vi "Lab Panel V4.87.vi"() -> ()   [LabVIEW 2013] (continued)
                      tunnel: w2786 -> [_ w2799]
                      tunnel: w2785 -> [_ w2798]
                      tunnel: w2784 -> [_ w2797]
                      frame False {
                      }
                      frame True {
                        n1475 = stacked-sequence {
                          tunnel: w2804 -> [w2808 _ _]
                          tunnel: w2803 -> [_ w2810 _]
                          tunnel: w2802 -> [_ _ _]
                          tunnel: w2801 -> [_ _ w2816]
                          tunnel: w2800 -> [_ _ w2815]
                          tunnel: w2799 -> [_ _ w2814]
                          tunnel: w2798 -> [_ _ w2813]
                          tunnel: w2797 -> [_ _ w2812]
                          frame #0 {
                            w2805 = FALSE
                            n1476 = local write "mail control"("END") -> ()
                            n1477 = Bundle(cluster=w2808) -> (w2807:T4)  [unwired: 3 in]
                            n1478 = local write "DISP LAB01-1"(w2807) -> ()
                            n1479 = local write "O/I  LAB01-1"(w2805) -> ()
                            n1480 = local write "run lab01-1"(w2805) -> ()
                            n1481 = local write "RUN LAB01-1"(w2805) -> ()
                          }
                          frame #1 {
                            n1482 = TDMS Close(11:w2810) -> (0:w2809:errorcluster)  [unwired: 1 in, 1 out]
                            n1483 = local write "data file error"(w2809) -> ()
                          }
                          frame #2 {
                            n1484 = stacked-sequence {
                              tunnel: "LAB01-1" -> [w2818 w2820 _]
                              tunnel: w2816 -> [_ w2826 _]
                              tunnel: w2815 -> [_ w2825 _]
                              tunnel: w2814 -> [_ w2824 _]
                              tunnel: w2813 -> [_ w2823 _]
                              tunnel: w2812 -> [_ w2822 _]
                              frame #0 {
                                n1485 = call "sub vi - defrag tdms v1.vi"("panel id"=w2818) -> ("error out"=w2817:errorcluster)  [unwired: 10 in]
                                n1486 = local write "data file error"(w2817) -> ()
                              }
                              frame #1 {
                                n1487 = Bundle("STATUS"=w2826, "OUT SERVER ADDRESS"=w2825, "FROM ACCOUNT"=w2824, "Mail Test File To:"=w2823, "Mail Test Fail"=w2822) -> (w2819:T25)  [unwired: 1 in]
                                n1488 = call "Save data file to network drive v3.vi"("Input Cluster"=w2819, "panel id"=w2820) -> ("network file save error"=w2821:errorcluster)  [unwired: 8 in, 1 out]
                                n1489 = local write "data file error"(w2821) -> ()
                              }
                              frame #2 {
                              }
                            }
                          }
                        }
                      }
                    }
                  }
                }
              }
              frame #1 {
                # "LAB01-2"
                n1490 = local read "run lab01-2"() -> (w2831:bool)
                n1491 = case shown="True" w2831 {
                  tunnel: w2830 -> [_ w2835]
                  tunnel: w2829 -> [_ w2834]
                  tunnel: w2828 -> [_ w2833]
                  tunnel: w2827 -> [_ w2832]
                  frame False {
                  }
                  frame True {
                    n1492 = local read "DISP LAB01-2"() -> (w2843:T4)
                    n1493 = local read "TDMS LAB01-2"() -> (w2842:refnum<k34>)
                    n1494 = Unbundle(w2843) -> ("CYCLE"=w2837:dbl, "STATUS"=w2836:string)  [unwired: 1 out]
                    n1495 = Not Equal?(x=w2836, y="RUN") -> (x != y?=w2839:bool)
                    n1496 = Greater?(x=w2837, y=2.0) -> (0:w2840:bool)
                    n1497 = And(x=w2840, y=w2839) -> (x .and. y?=w2838:bool)
                    n1498 = case shown="True" w2838 {
                      tunnel: w2843 -> [_ w2852]
                      tunnel: w2842 -> [_ w2851]
                      tunnel: w2837 -> [_ w2850]
                      tunnel: w2836 -> [_ w2849]
                      tunnel: w2835 -> [_ w2848]
                      tunnel: w2834 -> [_ w2847]
                      tunnel: w2833 -> [_ w2846]
                      tunnel: w2832 -> [_ w2845]
                      frame False {
                      }
                      frame True {
                        n1499 = stacked-sequence {
                          tunnel: w2852 -> [w2855 _ _]
                          tunnel: w2851 -> [_ w2857 _]
                          tunnel: w2850 -> [_ _ _]
                          tunnel: w2849 -> [_ _ w2863]
                          tunnel: w2848 -> [_ _ w2862]
                          tunnel: w2847 -> [_ _ w2861]
                          tunnel: w2846 -> [_ _ w2860]
                          tunnel: w2845 -> [_ _ w2859]
                          frame #0 {
                            w2853 = FALSE
                            n1500 = local write "mail control"("END") -> ()
                            n1501 = Bundle(cluster=w2855) -> (w2856:T4)  [unwired: 3 in]
                            n1502 = local write "RUN LAB01-2"(w2853) -> ()
                            n1503 = local write "run lab01-2"(w2853) -> ()
                            n1504 = local write "O/I  LAB01-2"(w2853) -> ()
                            n1505 = local write "DISP LAB01-2"(w2856) -> ()
                          }
                          frame #1 {
                            n1506 = TDMS Close(11:w2857) -> (0:w2858:errorcluster)  [unwired: 1 in, 1 out]
                            n1507 = local write "data file error"(w2858) -> ()
                          }
                          frame #2 {
                            n1508 = stacked-sequence {
                              tunnel: "LAB01-2" -> [w2866 w2867]
                              tunnel: w2863 -> [_ w2872]
                              tunnel: w2862 -> [_ w2871]
                              tunnel: w2861 -> [_ w2870]
                              tunnel: w2860 -> [_ w2869]
                              tunnel: w2859 -> [_ w2868]
                              frame #0 {
                                n1509 = call "sub vi - defrag tdms v1.vi"("panel id"=w2866) -> ("error out"=w2865:errorcluster)  [unwired: 10 in]
                                n1510 = local write "data file error"(w2865) -> ()
                              }
                              frame #1 {
                                n1511 = Bundle("STATUS"=w2872, "OUT SERVER ADDRESS"=w2871, "FROM ACCOUNT"=w2870, "Mail Test File To:"=w2869, "Mail Test Fail"=w2868) -> (w2874:T25)  [unwired: 1 in]
                                n1512 = call "Save data file to network drive v3.vi"("Input Cluster"=w2874, "panel id"=w2867) -> ("network file save error"=w2873:errorcluster)  [unwired: 8 in, 1 out]
                                n1513 = local write "data file error"(w2873) -> ()
                              }
                            }
                          }
                        }
                      }
                    }
                  }
                }
              }
              frame #2 {
                # "LAB02-1"
                n1514 = local read "run lab02-1"() -> (w2879:bool)
                n1515 = case shown="True" w2879 {
                  tunnel: w2878 -> [_ w2883]
                  tunnel: w2877 -> [_ w2882]
                  tunnel: w2876 -> [_ w2881]
                  tunnel: w2875 -> [_ w2880]
                  frame False {
                  }
                  frame True {
                    n1516 = local read "DISP LAB02-1"() -> (w2891:T4)
                    n1517 = Unbundle(w2891) -> ("CYCLE"=w2887:dbl, "STATUS"=w2884:string)  [unwired: 1 out]
                    n1518 = local read "TDMS LAB02-1"() -> (w2890:refnum<k34>)
                    n1519 = Not Equal?(x=w2884, y="RUN") -> (x != y?=w2886:bool)
                    n1520 = Greater?(x=w2887, y=2.0) -> (0:w2888:bool)
                    n1521 = And(x=w2888, y=w2886) -> (x .and. y?=w2885:bool)
                    n1522 = case shown="True" w2885 {
                      tunnel: w2891 -> [_ w2899]
                      tunnel: w2890 -> [_ w2898]
                      tunnel: w2884 -> [_ w2897]
                      tunnel: w2883 -> [_ w2896]
                      tunnel: w2882 -> [_ w2895]
                      tunnel: w2881 -> [_ w2894]
                      tunnel: w2880 -> [_ w2893]
                      frame False {
                      }
                      frame True {
                        n1523 = stacked-sequence {
                          tunnel: w2899 -> [w2902 _ _]
                          tunnel: w2898 -> [_ w2904 _]
                          tunnel: w2897 -> [_ _ w2910]
                          tunnel: w2896 -> [_ _ w2909]
                          tunnel: w2895 -> [_ _ w2908]
                          tunnel: w2894 -> [_ _ w2907]
                          tunnel: w2893 -> [_ _ w2906]
                          frame #0 {
                            w2900 = FALSE
                            n1524 = local write "mail control"("END") -> ()
                            n1525 = Bundle(cluster=w2902) -> (w2903:T4)  [unwired: 3 in]
                            n1526 = local write "O/I  LAB02-1"(w2900) -> ()
                            n1527 = local write "RUN LAB02-1"(w2900) -> ()
                            n1528 = local write "run lab02-1"(w2900) -> ()
                            n1529 = local write "DISP LAB02-1"(w2903) -> ()
                          }
                          frame #1 {
                            n1530 = TDMS Close(11:w2904) -> (0:w2905:errorcluster)  [unwired: 1 in, 1 out]
                            n1531 = local write "data file error"(w2905) -> ()
                          }
                          frame #2 {
                            n1532 = stacked-sequence {
                              tunnel: "LAB02-1" -> [w2913 w2920]
                              tunnel: w2910 -> [_ w2918]
                              tunnel: w2909 -> [_ w2917]
                              tunnel: w2908 -> [_ w2916]
                              tunnel: w2907 -> [_ w2915]
                              tunnel: w2906 -> [_ w2914]
                              frame #0 {
                                n1533 = call "sub vi - defrag tdms v1.vi"("panel id"=w2913) -> ("error out"=w2912:errorcluster)  [unwired: 10 in]
                                n1534 = local write "data file error"(w2912) -> ()
                              }
                              frame #1 {
                                n1535 = Bundle("STATUS"=w2918, "OUT SERVER ADDRESS"=w2917, "FROM ACCOUNT"=w2916, "Mail Test File To:"=w2915, "Mail Test Fail"=w2914) -> (w2919:T25)  [unwired: 1 in]
                                n1536 = call "Save data file to network drive v3.vi"("Input Cluster"=w2919, "panel id"=w2920) -> ("network file save error"=w2921:errorcluster)  [unwired: 8 in, 1 out]
                                n1537 = local write "data file error"(w2921) -> ()
                              }
                            }
                          }
                        }
                      }
                    }
                  }
                }
              }
              frame #3 {
                # "LAB02-2"
                n1538 = local read "run lab02-2"() -> (w2926:bool)
                n1539 = case shown="True" w2926 {
                  tunnel: w2925 -> [_ w2930]
                  tunnel: w2924 -> [_ w2929]
                  tunnel: w2923 -> [_ w2928]
                  tunnel: w2922 -> [_ w2927]
                  frame False {
                  }
                  frame True {
                    n1540 = local read "DISP LAB02-2"() -> (w2938:T4)
                    n1541 = local read "TDMS LAB02-2"() -> (w2937:refnum<k34>)
                    n1542 = Unbundle(w2938) -> ("CYCLE"=w2934:dbl, "STATUS"=w2931:string)  [unwired: 1 out]
                    n1543 = Not Equal?(x=w2931, y="RUN") -> (x != y?=w2933:bool)
                    n1544 = Greater?(x=w2934, y=2.0) -> (0:w2935:bool)
                    n1545 = And(x=w2935, y=w2933) -> (x .and. y?=w2932:bool)
                    n1546 = case shown="True" w2932 {
                      tunnel: w2938 -> [_ w2946]
                      tunnel: w2937 -> [_ w2945]
                      tunnel: w2931 -> [_ w2944]
                      tunnel: w2930 -> [_ w2943]
                      tunnel: w2929 -> [_ w2942]
                      tunnel: w2928 -> [_ w2941]
                      tunnel: w2927 -> [_ w2940]
                      frame False {
                      }
                      frame True {
                        n1547 = stacked-sequence {
                          tunnel: w2946 -> [w2949 _ _]
                          tunnel: w2945 -> [_ w2951 _]
                          tunnel: w2944 -> [_ _ w2957]
                          tunnel: w2943 -> [_ _ w2956]
                          tunnel: w2942 -> [_ _ w2955]
                          tunnel: w2941 -> [_ _ w2954]
                          tunnel: w2940 -> [_ _ w2953]
                          frame #0 {
                            w2947 = FALSE
                            n1548 = local write "mail control"("END") -> ()
                            n1549 = Bundle(cluster=w2949) -> (w2950:T4)  [unwired: 3 in]
                            n1550 = local write "O/I  LAB02-2"(w2947) -> ()
                            n1551 = local write "run lab02-2"(w2947) -> ()
                            n1552 = local write "RUN LAB02-2"(w2947) -> ()
                            n1553 = local write "DISP LAB02-2"(w2950) -> ()
                          }
                          frame #1 {
                            n1554 = TDMS Close(11:w2951) -> (0:w2952:errorcluster)  [unwired: 1 in, 1 out]
                            n1555 = local write "data file error"(w2952) -> ()
                          }
                          frame #2 {
                            n1556 = stacked-sequence {
                              tunnel: "LAB02-2" -> [w2960 w2966]
                              tunnel: w2957 -> [_ w2965]
                              tunnel: w2956 -> [_ w2964]
                              tunnel: w2955 -> [_ w2963]
                              tunnel: w2954 -> [_ w2962]
                              tunnel: w2953 -> [_ w2961]
                              frame #0 {
                                n1557 = call "sub vi - defrag tdms v1.vi"("panel id"=w2960) -> ("error out"=w2959:errorcluster)  [unwired: 10 in]
                                n1558 = local write "data file error"(w2959) -> ()
                              }
                              frame #1 {
                                n1559 = Bundle("STATUS"=w2965, "OUT SERVER ADDRESS"=w2964, "FROM ACCOUNT"=w2963, "Mail Test File To:"=w2962, "Mail Test Fail"=w2961) -> (w2968:T25)  [unwired: 1 in]
                                n1560 = call "Save data file to network drive v3.vi"("Input Cluster"=w2968, "panel id"=w2966) -> ("network file save error"=w2967:errorcluster)  [unwired: 8 in, 1 out]
                                n1561 = local write "data file error"(w2967) -> ()
                              }
                            }
                          }
                        }
                      }
                    }
                  }
                }
              }
              frame #4 {
                # "LAB03-1"
                n1562 = local read "run lab03-1"() -> (w2973:bool)
                n1563 = case shown="True" w2973 {
                  tunnel: w2972 -> [_ w2977]
                  tunnel: w2971 -> [_ w2976]
                  tunnel: w2970 -> [_ w2975]
                  tunnel: w2969 -> [_ w2974]
                  frame False {
                  }
                  frame True {
                    n1564 = local read "DISP LAB03-1"() -> (w2985:T4)
                    n1565 = local read "TDMS LAB03-1"() -> (w2984:refnum<k34>)
                    n1566 = Unbundle(w2985) -> ("CYCLE"=w2981:dbl, "STATUS"=w2978:string)  [unwired: 1 out]
                    n1567 = Not Equal?(x=w2978, y="RUN") -> (x != y?=w2980:bool)
                    n1568 = Greater?(x=w2981, y=2.0) -> (0:w2982:bool)
                    n1569 = And(x=w2982, y=w2980) -> (x .and. y?=w2979:bool)
                    n1570 = case shown="True" w2979 {
                      tunnel: w2985 -> [_ w2993]
                      tunnel: w2984 -> [_ w2992]
                      tunnel: w2978 -> [_ w2991]
                      tunnel: w2977 -> [_ w2990]
                      tunnel: w2976 -> [_ w2989]
                      tunnel: w2975 -> [_ w2988]
                      tunnel: w2974 -> [_ w2987]
                      frame False {
                      }
                      frame True {
                        n1571 = stacked-sequence {
                          tunnel: w2993 -> [w2996 _ _]
                          tunnel: w2992 -> [_ w2998 _]
                          tunnel: w2991 -> [_ _ w3004]
                          tunnel: w2990 -> [_ _ w3003]
                          tunnel: w2989 -> [_ _ w3002]
                          tunnel: w2988 -> [_ _ w3001]
                          tunnel: w2987 -> [_ _ w3000]
                          frame #0 {
                            w2994 = FALSE
                            n1572 = local write "mail control"("END") -> ()
                            n1573 = Bundle(cluster=w2996) -> (w2997:T4)  [unwired: 3 in]
                            n1574 = local write "O/I  LAB03-1"(w2994) -> ()
                            n1575 = local write "run lab03-1"(w2994) -> ()
                            n1576 = local write "RUN LAB03-1"(w2994) -> ()
                            n1577 = local write "DISP LAB03-1"(w2997) -> ()
                          }
                          frame #1 {
                            n1578 = TDMS Close(11:w2998) -> (0:w2999:errorcluster)  [unwired: 1 in, 1 out]
                            n1579 = local write "data file error"(w2999) -> ()
                          }
                          frame #2 {
                            n1580 = stacked-sequence {
                              tunnel: "LAB03-1" -> [w3007 w3013]
                              tunnel: w3004 -> [_ w3012]
                              tunnel: w3003 -> [_ w3011]
                              tunnel: w3002 -> [_ w3010]
                              tunnel: w3001 -> [_ w3009]
                              tunnel: w3000 -> [_ w3008]
                              frame #0 {
                                n1581 = call "sub vi - defrag tdms v1.vi"("panel id"=w3007) -> ("error out"=w3006:errorcluster)  [unwired: 10 in]
                                n1582 = local write "data file error"(w3006) -> ()
                              }
                              frame #1 {
                                n1583 = Bundle("STATUS"=w3012, "OUT SERVER ADDRESS"=w3011, "FROM ACCOUNT"=w3010, "Mail Test File To:"=w3009, "Mail Test Fail"=w3008) -> (w3015:T25)  [unwired: 1 in]
                                n1584 = call "Save data file to network drive v3.vi"("Input Cluster"=w3015, "panel id"=w3013) -> ("network file save error"=w3014:errorcluster)  [unwired: 8 in, 1 out]
                                n1585 = local write "data file error"(w3014) -> ()
                              }
                            }
                          }
                        }
                      }
                    }
                  }
                }
              }
              frame #5 {
                # "LAB03-2"
                n1586 = local read "run lab03-2"() -> (w3020:bool)
                n1587 = case shown="True" w3020 {
                  tunnel: w3019 -> [_ w3024]
                  tunnel: w3018 -> [_ w3023]
                  tunnel: w3017 -> [_ w3022]
                  tunnel: w3016 -> [_ w3021]
                  frame False {
                  }
                  frame True {
                    n1588 = local read "DISP LAB03-2"() -> (w3032:T4)
                    n1589 = Unbundle(w3032) -> ("CYCLE"=w3028:dbl, "STATUS"=w3025:string)  [unwired: 1 out]
                    n1590 = local read "TDMS LAB03-2"() -> (w3031:refnum<k34>)
                    n1591 = Not Equal?(x=w3025, y="RUN") -> (x != y?=w3027:bool)
                    n1592 = Greater?(x=w3028, y=2.0) -> (0:w3029:bool)
                    n1593 = And(x=w3029, y=w3027) -> (x .and. y?=w3026:bool)
                    n1594 = case shown="True" w3026 {
                      tunnel: w3032 -> [_ w3040]
                      tunnel: w3031 -> [_ w3039]
                      tunnel: w3025 -> [_ w3038]
                      tunnel: w3024 -> [_ w3037]
                      tunnel: w3023 -> [_ w3036]
                      tunnel: w3022 -> [_ w3035]
                      tunnel: w3021 -> [_ w3034]
                      frame False {
                      }
                      frame True {
                        n1595 = stacked-sequence {
                          tunnel: w3040 -> [w3043 _ _]
                          tunnel: w3039 -> [_ w3045 _]
                          tunnel: w3038 -> [_ _ w3051]
                          tunnel: w3037 -> [_ _ w3050]
                          tunnel: w3036 -> [_ _ w3049]
                          tunnel: w3035 -> [_ _ w3048]
                          tunnel: w3034 -> [_ _ w3047]
                          frame #0 {
                            w3041 = FALSE
                            n1596 = local write "mail control"("END") -> ()
                            n1597 = Bundle(cluster=w3043) -> (w3044:T4)  [unwired: 3 in]
                            n1598 = local write "RUN LAB03-2"(w3041) -> ()
                            n1599 = local write "O/I  LAB03-2"(w3041) -> ()
                            n1600 = local write "DISP LAB03-2"(w3044) -> ()
                            n1601 = local write "run lab03-2"(w3041) -> ()
                          }
                          frame #1 {
                            n1602 = TDMS Close(11:w3045) -> (0:w3046:errorcluster)  [unwired: 1 in, 1 out]
                            n1603 = local write "data file error"(w3046) -> ()
                          }
                          frame #2 {
                            n1604 = stacked-sequence {
                              tunnel: "LAB03-2" -> [w3054 w3055]
                              tunnel: w3051 -> [_ w3060]
                              tunnel: w3050 -> [_ w3059]
                              tunnel: w3049 -> [_ w3058]
                              tunnel: w3048 -> [_ w3057]
                              tunnel: w3047 -> [_ w3056]
                              frame #0 {
                                n1605 = call "sub vi - defrag tdms v1.vi"("panel id"=w3054) -> ("error out"=w3053:errorcluster)  [unwired: 10 in]
                                n1606 = local write "data file error"(w3053) -> ()
                              }
                              frame #1 {
                                n1607 = Bundle("STATUS"=w3060, "OUT SERVER ADDRESS"=w3059, "FROM ACCOUNT"=w3058, "Mail Test File To:"=w3057, "Mail Test Fail"=w3056) -> (w3062:T25)  [unwired: 1 in]
                                n1608 = call "Save data file to network drive v3.vi"("Input Cluster"=w3062, "panel id"=w3055) -> ("network file save error"=w3061:errorcluster)  [unwired: 8 in, 1 out]
                                n1609 = local write "data file error"(w3061) -> ()
                              }
                            }
                          }
                        }
                      }
                    }
                  }
                }
              }
              frame #6 {
                # "LAB04-1"
                n1610 = local read "run lab04-1"() -> (w3067:bool)
                n1611 = case shown="True" w3067 {
                  tunnel: w3066 -> [_ w3071]
                  tunnel: w3065 -> [_ w3070]
                  tunnel: w3064 -> [_ w3069]
                  tunnel: w3063 -> [_ w3068]
                  frame False {
                  }
                  frame True {
                    n1612 = local read "DISP LAB04-1"() -> (w3079:T4)
                    n1613 = Unbundle(w3079) -> ("CYCLE"=w3075:dbl, "STATUS"=w3072:string)  [unwired: 1 out]
                    n1614 = local read "TDMS LAB04-1"() -> (w3078:refnum<k34>)
                    n1615 = Not Equal?(x=w3072, y="RUN") -> (x != y?=w3074:bool)
                    n1616 = Greater?(x=w3075, y=2.0) -> (0:w3076:bool)
                    n1617 = And(x=w3076, y=w3074) -> (x .and. y?=w3073:bool)
                    n1618 = case shown="True" w3073 {
                      tunnel: w3079 -> [_ w3087]
                      tunnel: w3078 -> [_ w3086]
                      tunnel: w3072 -> [_ w3085]
                      tunnel: w3071 -> [_ w3084]
                      tunnel: w3070 -> [_ w3083]
                      tunnel: w3069 -> [_ w3082]
                      tunnel: w3068 -> [_ w3081]
                      frame False {
                      }
                      frame True {
                        n1619 = stacked-sequence {
                          tunnel: w3087 -> [w3090 _ _]
                          tunnel: w3086 -> [_ w3092 _]
                          tunnel: w3085 -> [_ _ w3098]
                          tunnel: w3084 -> [_ _ w3097]
                          tunnel: w3083 -> [_ _ w3096]
                          tunnel: w3082 -> [_ _ w3095]
                          tunnel: w3081 -> [_ _ w3094]
                          frame #0 {
                            w3088 = FALSE
                            n1620 = local write "mail control"("END") -> ()
                            n1621 = Bundle(cluster=w3090) -> (w3091:T4)  [unwired: 3 in]
                            n1622 = local write "RUN LAB04-1"(w3088) -> ()
                            n1623 = local write "O/I  LAB04-1"(w3088) -> ()
                            n1624 = local write "run lab04-1"(w3088) -> ()
                            n1625 = local write "DISP LAB04-1"(w3091) -> ()
                          }
                          frame #1 {
                            n1626 = TDMS Close(11:w3092) -> (0:w3093:errorcluster)  [unwired: 1 in, 1 out]
                            n1627 = local write "data file error"(w3093) -> ()
                          }
                          frame #2 {
                            n1628 = stacked-sequence {
                              tunnel: "LAB04-1" -> [w3101 w3102]
                              tunnel: w3098 -> [_ w3107]
                              tunnel: w3097 -> [_ w3106]
                              tunnel: w3096 -> [_ w3105]
                              tunnel: w3095 -> [_ w3104]
                              tunnel: w3094 -> [_ w3103]
                              frame #0 {
                                n1629 = call "sub vi - defrag tdms v1.vi"("panel id"=w3101) -> ("error out"=w3100:errorcluster)  [unwired: 10 in]
                                n1630 = local write "data file error"(w3100) -> ()
                              }
                              frame #1 {
                                n1631 = Bundle("STATUS"=w3107, "OUT SERVER ADDRESS"=w3106, "FROM ACCOUNT"=w3105, "Mail Test File To:"=w3104, "Mail Test Fail"=w3103) -> (w3109:T25)  [unwired: 1 in]
                                n1632 = call "Save data file to network drive v3.vi"("Input Cluster"=w3109, "panel id"=w3102) -> ("network file save error"=w3108:errorcluster)  [unwired: 8 in, 1 out]
                                n1633 = local write "data file error"(w3108) -> ()
                              }
                            }
                          }
                        }
                      }
                    }
                  }
                }
              }
              frame #7 {
                # "LAB04-2"
                n1634 = local read "run lab04-2"() -> (w3114:bool)
                n1635 = case shown="True" w3114 {
                  tunnel: w3113 -> [_ w3118]
                  tunnel: w3112 -> [_ w3117]
                  tunnel: w3111 -> [_ w3116]
                  tunnel: w3110 -> [_ w3115]
                  frame False {
                  }
                  frame True {
                    n1636 = local read "DISP LAB04-2"() -> (w3126:T4)
                    n1637 = Unbundle(w3126) -> ("CYCLE"=w3122:dbl, "STATUS"=w3119:string)  [unwired: 1 out]
                    n1638 = Not Equal?(x=w3119, y="RUN") -> (x != y?=w3121:bool)
                    n1639 = local read "TDMS LAB04-2"() -> (w3125:refnum<k34>)
                    n1640 = Greater?(x=w3122, y=2.0) -> (0:w3123:bool)
                    n1641 = And(x=w3123, y=w3121) -> (x .and. y?=w3120:bool)
                    n1642 = case shown="True" w3120 {
                      tunnel: w3126 -> [_ w3134]
                      tunnel: w3125 -> [_ w3133]
                      tunnel: w3119 -> [_ w3132]
                      tunnel: w3118 -> [_ w3131]
                      tunnel: w3117 -> [_ w3130]
                      tunnel: w3116 -> [_ w3129]
                      tunnel: w3115 -> [_ w3128]
                      frame False {
                      }
                      frame True {
                        n1643 = stacked-sequence {
                          tunnel: w3134 -> [w3137 _ _]
                          tunnel: w3133 -> [_ w3139 _]
                          tunnel: w3132 -> [_ _ w3145]
                          tunnel: w3131 -> [_ _ w3144]
                          tunnel: w3130 -> [_ _ w3143]
                          tunnel: w3129 -> [_ _ w3142]
                          tunnel: w3128 -> [_ _ w3141]
                          frame #0 {
                            w3135 = FALSE
                            n1644 = local write "mail control"("END") -> ()
                            n1645 = Bundle(cluster=w3137) -> (w3138:T4)  [unwired: 3 in]
                            n1646 = local write "O/I  LAB04-2"(w3135) -> ()
                            n1647 = local write "RUN LAB04-2"(w3135) -> ()
                            n1648 = local write "run lab04-2"(w3135) -> ()
                            n1649 = local write "DISP LAB04-2"(w3138) -> ()
                          }
                          frame #1 {
                            n1650 = TDMS Close(11:w3139) -> (0:w3140:errorcluster)  [unwired: 1 in, 1 out]
                            n1651 = local write "data file error"(w3140) -> ()
                          }
                          frame #2 {
                            n1652 = stacked-sequence {
                              tunnel: "LAB04-2" -> [w3148 w3149]
                              tunnel: w3145 -> [_ w3154]
                              tunnel: w3144 -> [_ w3153]
                              tunnel: w3143 -> [_ w3152]
                              tunnel: w3142 -> [_ w3151]
                              tunnel: w3141 -> [_ w3150]
                              frame #0 {
                                n1653 = call "sub vi - defrag tdms v1.vi"("panel id"=w3148) -> ("error out"=w3147:errorcluster)  [unwired: 10 in]
                                n1654 = local write "data file error"(w3147) -> ()
                              }
                              frame #1 {
                                n1655 = Bundle("STATUS"=w3154, "OUT SERVER ADDRESS"=w3153, "FROM ACCOUNT"=w3152, "Mail Test File To:"=w3151, "Mail Test Fail"=w3150) -> (w3156:T25)  [unwired: 1 in]
                                n1656 = call "Save data file to network drive v3.vi"("Input Cluster"=w3156, "panel id"=w3149) -> ("network file save error"=w3155:errorcluster)  [unwired: 8 in, 1 out]
                                n1657 = local write "data file error"(w3155) -> ()
                              }
                            }
                          }
                        }
                      }
                    }
                  }
                }
              }
              frame #8 {
                # "LAB05-1"
                n1658 = local read "run lab05-1"() -> (w3161:bool)
                n1659 = case shown="True" w3161 {
                  tunnel: w3160 -> [_ w3165]
                  tunnel: w3159 -> [_ w3164]
                  tunnel: w3158 -> [_ w3163]
                  tunnel: w3157 -> [_ w3162]
                  frame False {
                  }
                  frame True {
                    n1660 = local read "DISP LAB05-1"() -> (w3173:T4)
                    n1661 = Unbundle(w3173) -> ("CYCLE"=w3169:dbl, "STATUS"=w3166:string)  [unwired: 1 out]
                    n1662 = Not Equal?(x=w3166, y="RUN") -> (x != y?=w3168:bool)
                    n1663 = local read "TDMS LAB05-1"() -> (w3172:refnum<k34>)
                    n1664 = Greater?(x=w3169, y=2.0) -> (0:w3170:bool)
                    n1665 = And(x=w3170, y=w3168) -> (x .and. y?=w3167:bool)
                    n1666 = case shown="True" w3167 {
                      tunnel: w3173 -> [_ w3181]
                      tunnel: w3172 -> [_ w3180]
                      tunnel: w3166 -> [_ w3179]
                      tunnel: w3165 -> [_ w3178]
                      tunnel: w3164 -> [_ w3177]
                      tunnel: w3163 -> [_ w3176]
                      tunnel: w3162 -> [_ w3175]
                      frame False {
                      }
                      frame True {
                        n1667 = stacked-sequence {
                          tunnel: w3181 -> [w3184 _ _]
                          tunnel: w3180 -> [_ w3186 _]
                          tunnel: w3179 -> [_ _ w3192]
                          tunnel: w3178 -> [_ _ w3191]
                          tunnel: w3177 -> [_ _ w3190]
                          tunnel: w3176 -> [_ _ w3189]
                          tunnel: w3175 -> [_ _ w3188]
                          frame #0 {
                            w3182 = FALSE
                            n1668 = local write "mail control"("END") -> ()
                            n1669 = Bundle(cluster=w3184) -> (w3185:T4)  [unwired: 3 in]
                            n1670 = local write "O/I  LAB05-1"(w3182) -> ()
                            n1671 = local write "RUN LAB05-1"(w3182) -> ()
                            n1672 = local write "run lab05-1"(w3182) -> ()
                            n1673 = local write "DISP LAB05-1"(w3185) -> ()
                          }
                          frame #1 {
                            n1674 = TDMS Close(11:w3186) -> (0:w3187:errorcluster)  [unwired: 1 in, 1 out]
                            n1675 = local write "data file error"(w3187) -> ()
                          }
                          frame #2 {
                            n1676 = stacked-sequence {
                              tunnel: "LAB05-1" -> [w3195 w3201]
                              tunnel: w3192 -> [_ w3200]
                              tunnel: w3191 -> [_ w3199]
                              tunnel: w3190 -> [_ w3198]
                              tunnel: w3189 -> [_ w3197]
                              tunnel: w3188 -> [_ w3196]
                              frame #0 {
                                n1677 = call "sub vi - defrag tdms v1.vi"("panel id"=w3195) -> ("error out"=w3194:errorcluster)  [unwired: 10 in]
                                n1678 = local write "data file error"(w3194) -> ()
                              }
                              frame #1 {
                                n1679 = Bundle("STATUS"=w3200, "OUT SERVER ADDRESS"=w3199, "FROM ACCOUNT"=w3198, "Mail Test File To:"=w3197, "Mail Test Fail"=w3196) -> (w3203:T25)  [unwired: 1 in]
                                n1680 = call "Save data file to network drive v3.vi"("Input Cluster"=w3203, "panel id"=w3201) -> ("network file save error"=w3202:errorcluster)  [unwired: 8 in, 1 out]
                                n1681 = local write "data file error"(w3202) -> ()
                              }
                            }
                          }
                        }
                      }
                    }
                  }
                }
              }
              frame #9 {
                # "LAB05-2"
                n1682 = local read "run lab05-2"() -> (w3208:bool)
                n1683 = case shown="True" w3208 {
                  tunnel: w3207 -> [_ w3212]
                  tunnel: w3206 -> [_ w3211]
                  tunnel: w3205 -> [_ w3210]
                  tunnel: w3204 -> [_ w3209]
                  frame False {
                  }
                  frame True {
                    n1684 = local read "DISP LAB05-2"() -> (w3220:T4)
                    n1685 = Unbundle(w3220) -> ("CYCLE"=w3216:dbl, "STATUS"=w3213:string)  [unwired: 1 out]
                    n1686 = Not Equal?(x=w3213, y="RUN") -> (x != y?=w3215:bool)
                    n1687 = local read "TDMS LAB05-2"() -> (w3219:refnum<k34>)
                    n1688 = Greater?(x=w3216, y=2.0) -> (0:w3217:bool)
                    n1689 = And(x=w3217, y=w3215) -> (x .and. y?=w3214:bool)
                    n1690 = case shown="True" w3214 {
                      tunnel: w3220 -> [_ w3228]
                      tunnel: w3219 -> [_ w3227]
                      tunnel: w3213 -> [_ w3226]
                      tunnel: w3212 -> [_ w3225]
                      tunnel: w3211 -> [_ w3224]
                      tunnel: w3210 -> [_ w3223]
                      tunnel: w3209 -> [_ w3222]
                      frame False {
                      }
                      frame True {
                        n1691 = stacked-sequence {
                          tunnel: w3228 -> [w3231 _ _]
                          tunnel: w3227 -> [_ w3233 _]
                          tunnel: w3226 -> [_ _ w3239]
                          tunnel: w3225 -> [_ _ w3238]
                          tunnel: w3224 -> [_ _ w3237]
                          tunnel: w3223 -> [_ _ w3236]
                          tunnel: w3222 -> [_ _ w3235]
                          frame #0 {
                            w3229 = FALSE
                            n1692 = local write "mail control"("END") -> ()
                            n1693 = Bundle(cluster=w3231) -> (w3232:T4)  [unwired: 3 in]
                            n1694 = local write "RUN LAB05-2"(w3229) -> ()
                            n1695 = local write "O/I  LAB05-2"(w3229) -> ()
                            n1696 = local write "run lab05-2"(w3229) -> ()
                            n1697 = local write "DISP LAB05-2"(w3232) -> ()
                          }
                          frame #1 {
                            n1698 = TDMS Close(11:w3233) -> (0:w3234:errorcluster)  [unwired: 1 in, 1 out]
                            n1699 = local write "data file error"(w3234) -> ()
                          }
                          frame #2 {
                            n1700 = stacked-sequence {
                              tunnel: "LAB05-2" -> [w3242 w3248]
                              tunnel: w3239 -> [_ w3247]
                              tunnel: w3238 -> [_ w3246]
                              tunnel: w3237 -> [_ w3245]
                              tunnel: w3236 -> [_ w3244]
                              tunnel: w3235 -> [_ w3243]
                              frame #0 {
                                n1701 = call "sub vi - defrag tdms v1.vi"("panel id"=w3242) -> ("error out"=w3241:errorcluster)  [unwired: 10 in]
                                n1702 = local write "data file error"(w3241) -> ()
                              }
                              frame #1 {
                                n1703 = Bundle("STATUS"=w3247, "OUT SERVER ADDRESS"=w3246, "FROM ACCOUNT"=w3245, "Mail Test File To:"=w3244, "Mail Test Fail"=w3243) -> (w3250:T25)  [unwired: 1 in]
                                n1704 = call "Save data file to network drive v3.vi"("Input Cluster"=w3250, "panel id"=w3248) -> ("network file save error"=w3249:errorcluster)  [unwired: 8 in, 1 out]
                                n1705 = local write "data file error"(w3249) -> ()
                              }
                            }
                          }
                        }
                      }
                    }
                  }
                }
              }
            }
            n1706 = local read "Network Directory"() -> (w2764:path)
            n1707 = global write "Global 1.vi" "Network Drive"(w2764) -> ()
          }
          frame #7 {
            # "disable functions"
            n1708 = stacked-sequence {
              tunnel: w3260 -> [w3274 _ w3331]
              tunnel: w3259 -> [w3269 _ w3330]
              tunnel: w3258 -> [w3268 _ w3329]
              tunnel: w3257 -> [w3266 _ w3328]
              tunnel: w3256 -> [w3267 _ w3327]
              tunnel: w3255 -> [_ w3291 w3326]
              tunnel: w3254 -> [_ w3292 w3325]
              tunnel: w3253 -> [_ w3293 w3324]
              tunnel: w3252 -> [_ w3294 w3323]
              tunnel: w3251 -> [_ w3295 w3322]
              frame #0 {
                n1709 = Select(t=2, s=w3266, f=0) -> (s? t:f=w3262:i32)
                n1710 = Select(t=2, s=w3268, f=0) -> (s? t:f=w3263:i32)
                n1711 = Select(t=2, s=w3267, f=0) -> (s? t:f=w3261:i32)
                n1712 = Select(t=2, s=w3274, f=0) -> (s? t:f=w3265:i32)
                n1713 = Select(t=2, s=w3269, f=0) -> (s? t:f=w3264:i32)
                n1714 = property on="SELECT LAB02-2" class="RadioBtnsControl (strict)"("DisabledEnum"=w3262) -> ()  [unwired: 2 in, 2 out]
                n1715 = property on="SELECT LAB02-1" class="RadioBtnsControl (strict)"("DisabledEnum"=w3263) -> ()  [unwired: 2 in, 2 out]
                n1716 = property on="SELECT LAB03-1" class="RadioBtnsControl (strict)"("DisabledEnum"=w3261) -> ()  [unwired: 2 in, 2 out]
                n1717 = property on="SELECT LAB01-1" class="RadioBtnsControl (strict)"("DisabledEnum"=w3265) -> ()  [unwired: 2 in, 2 out]
                n1718 = property on="SELECT LAB01-2" class="RadioBtnsControl (strict)"("DisabledEnum"=w3264) -> ()  [unwired: 2 in, 2 out]
                n1719 = Not(x=w3274) -> (.not. x?=w3275:bool)
                n1720 = property on="RESULT LAB01-1" class="Bool (strict)"("Visible"=w3275) -> ()  [unwired: 2 in, 2 out]
                n1721 = Not(x=w3269) -> (.not. x?=w3273:bool)
                n1722 = Not(x=w3268) -> (.not. x?=w3272:bool)
                n1723 = Not(x=w3266) -> (.not. x?=w3271:bool)
                n1724 = property on="RESULT LAB01-2" class="Bool (strict)"("Visible"=w3273) -> ()  [unwired: 2 in, 2 out]
                n1725 = Not(x=w3267) -> (.not. x?=w3270:bool)
                n1726 = property on="RESULT LAB02-1" class="Bool (strict)"("Visible"=w3272) -> ()  [unwired: 2 in, 2 out]
                n1727 = property on="RESULT LAB02-2" class="Bool (strict)"("Visible"=w3271) -> ()  [unwired: 2 in, 2 out]
                n1728 = property on="RESULT LAB03-1" class="Bool (strict)"("Visible"=w3270) -> ()  [unwired: 2 in, 2 out]
                n1729 = property on="SET LAB01-1" class="Clust (strict)"("DisabledEnum"=w3265) -> ()  [unwired: 2 in, 2 out]
                n1730 = property on="SET LAB01-2" class="Clust (strict)"("DisabledEnum"=w3264) -> ()  [unwired: 2 in, 2 out]
                n1731 = property on="SET LAB02-1" class="Clust (strict)"("DisabledEnum"=w3263) -> ()  [unwired: 2 in, 2 out]
                n1732 = property on="SET LAB02-2" class="Clust (strict)"("DisabledEnum"=w3262) -> ()  [unwired: 2 in, 2 out]
                n1733 = property on="SET LAB03-1" class="Clust (strict)"("DisabledEnum"=w3261) -> ()  [unwired: 2 in, 2 out]
                n1734 = property on="O/I  LAB01-1" class="Bool (strict)"("DisabledEnum"=w3265) -> ()  [unwired: 2 in, 2 out]
                n1735 = property on="O/I  LAB01-2" class="Bool (strict)"("DisabledEnum"=w3264) -> ()  [unwired: 2 in, 2 out]
                n1736 = property on="O/I  LAB02-1" class="Bool (strict)"("DisabledEnum"=w3263) -> ()  [unwired: 2 in, 2 out]
                n1737 = property on="O/I  LAB02-2" class="Bool (strict)"("DisabledEnum"=w3262) -> ()  [unwired: 2 in, 2 out]
                n1738 = property on="O/I  LAB03-1" class="Bool (strict)"("DisabledEnum"=w3261) -> ()  [unwired: 2 in, 2 out]
              }
              frame #1 {
                n1739 = Select(t=2, s=w3295, f=0) -> (s? t:f=w3286:i32)
                n1740 = Select(t=2, s=w3294, f=0) -> (s? t:f=w3287:i32)
                n1741 = Select(t=2, s=w3291, f=0) -> (s? t:f=w3290:i32)
                n1742 = Select(t=2, s=w3292, f=0) -> (s? t:f=w3289:i32)
                n1743 = Select(t=2, s=w3293, f=0) -> (s? t:f=w3288:i32)
                n1744 = property on="SELECT LAB05-2" class="RadioBtnsControl (strict)"("DisabledEnum"=w3286) -> ()  [unwired: 2 in, 2 out]
                n1745 = property on="SELECT LAB05-1" class="RadioBtnsControl (strict)"("DisabledEnum"=w3287) -> ()  [unwired: 2 in, 2 out]
                n1746 = property on="SELECT LAB03-2" class="RadioBtnsControl (strict)"("DisabledEnum"=w3290) -> ()  [unwired: 2 in, 2 out]
                n1747 = property on="SELECT LAB04-1" class="RadioBtnsControl (strict)"("DisabledEnum"=w3289) -> ()  [unwired: 2 in, 2 out]
                n1748 = property on="SELECT LAB04-2" class="RadioBtnsControl (strict)"("DisabledEnum"=w3288) -> ()  [unwired: 2 in, 2 out]
                n1749 = property on="SET LAB05-2" class="Clust (strict)"("DisabledEnum"=w3286) -> ()  [unwired: 2 in, 2 out]
                n1750 = property on="SET LAB05-1" class="Clust (strict)"("DisabledEnum"=w3287) -> ()  [unwired: 2 in, 2 out]
                n1751 = property on="SET LAB03-2" class="Clust (strict)"("DisabledEnum"=w3290) -> ()  [unwired: 2 in, 2 out]
                n1752 = property on="SET LAB04-1" class="Clust (strict)"("DisabledEnum"=w3289) -> ()  [unwired: 2 in, 2 out]
                n1753 = property on="SET LAB04-2" class="Clust (strict)"("DisabledEnum"=w3288) -> ()  [unwired: 2 in, 2 out]
                n1754 = property on="O/I  LAB05-2" class="Bool (strict)"("DisabledEnum"=w3286) -> ()  [unwired: 2 in, 2 out]
                n1755 = property on="O/I  LAB05-1" class="Bool (strict)"("DisabledEnum"=w3287) -> ()  [unwired: 2 in, 2 out]
                n1756 = property on="O/I  LAB04-1" class="Bool (strict)"("DisabledEnum"=w3289) -> ()  [unwired: 2 in, 2 out]
                n1757 = property on="O/I  LAB04-2" class="Bool (strict)"("DisabledEnum"=w3288) -> ()  [unwired: 2 in, 2 out]
                n1758 = property on="O/I  LAB03-2" class="Bool (strict)"("DisabledEnum"=w3290) -> ()  [unwired: 2 in, 2 out]
                n1759 = Not(x=w3295) -> (.not. x?=w3296:bool)
                n1760 = Not(x=w3294) -> (.not. x?=w3297:bool)
                n1761 = Not(x=w3293) -> (.not. x?=w3298:bool)
                n1762 = property on="RESULT LAB05-2" class="Bool (strict)"("Visible"=w3296) -> ()  [unwired: 2 in, 2 out]
                n1763 = property on="RESULT LAB05-1" class="Bool (strict)"("Visible"=w3297) -> ()  [unwired: 2 in, 2 out]
                n1764 = Not(x=w3292) -> (.not. x?=w3299:bool)
                n1765 = property on="RESULT LAB04-2" class="Bool (strict)"("Visible"=w3298) -> ()  [unwired: 2 in, 2 out]
                n1766 = Not(x=w3291) -> (.not. x?=w3300:bool)
                n1767 = property on="RESULT LAB04-1" class="Bool (strict)"("Visible"=w3299) -> ()  [unwired: 2 in, 2 out]
                n1768 = property on="RESULT LAB03-2" class="Bool (strict)"("Visible"=w3300) -> ()  [unwired: 2 in, 2 out]
              }
              frame #2 {
                # "disable calibrate if any test running"
                n1769 = Or(x=w3323, y=w3322) -> (x .or. y?=w3316:bool)
                n1770 = Or(x=w3325, y=w3324) -> (x .or. y?=w3318:bool)
                n1771 = Or(x=w3329, y=w3328) -> (x .or. y?=w3320:bool)
                n1772 = Or(x=w3327, y=w3326) -> (x .or. y?=w3319:bool)
                n1773 = Or(x=w3331, y=w3330) -> (x .or. y?=w3321:bool)
                n1774 = Or(x=w3319, y=w3318) -> (x .or. y?=w3317:bool)
                n1775 = Or(x=w3321, y=w3320) -> (x .or. y?=w3315:bool)
                n1776 = Or(x=w3317, y=w3316) -> (x .or. y?=w3314:bool)
                n1777 = Or(x=w3315, y=w3314) -> (x .or. y?=w3313:bool)
                n1778 = case shown="False" w3313 {
                  tunnel: [0 2] -> w3312
                  frame False {
                  }
                  frame True {
                  }
                }
                n1779 = property on="JIG TEST" class="Clust (strict)"("DisabledEnum"=w3312) -> ()  [unwired: 2 in, 2 out]
                n1780 = property on="Network Directory" class="Path"("DisabledEnum"=w3312) -> ()  [unwired: 2 in, 2 out]
                n1781 = property on="MAIL SETTINGS" class="Clust (strict)"("DisabledEnum"=w3312) -> ()  [unwired: 2 in, 2 out]
                n1782 = property on="SET (cal)" class="Bool (strict)"("DisabledEnum"=w3312) -> ()  [unwired: 2 in, 2 out]
                n1783 = property on="ADMIN" class="Bool (strict)"("DisabledEnum"=0) -> ()  [unwired: 2 in, 2 out]
              }
            }
          }
          frame #8 {
            # "drive jigs"
            n1784 = stacked-sequence {
              frame #0 {
                # "jig on"
                n1785 = local read "jig cycle"() -> (w3339:dbl)
